vi "Host-Top-Level.vi"() -> ()   [LabVIEW 2017]
uses:
  <vilib>/rvi/interface/nirviMethod/nirviMethod.xnode
  <vilib>/FPGAPlugInAG/Dynamic/niLvFpga_Run_Dynamic.vi
panel:
  in  "Device address":string
  in  "Bitfile path":path
  in  "error in":errorcluster
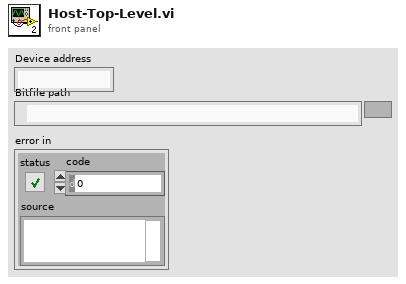
[diagram p1: front panel]
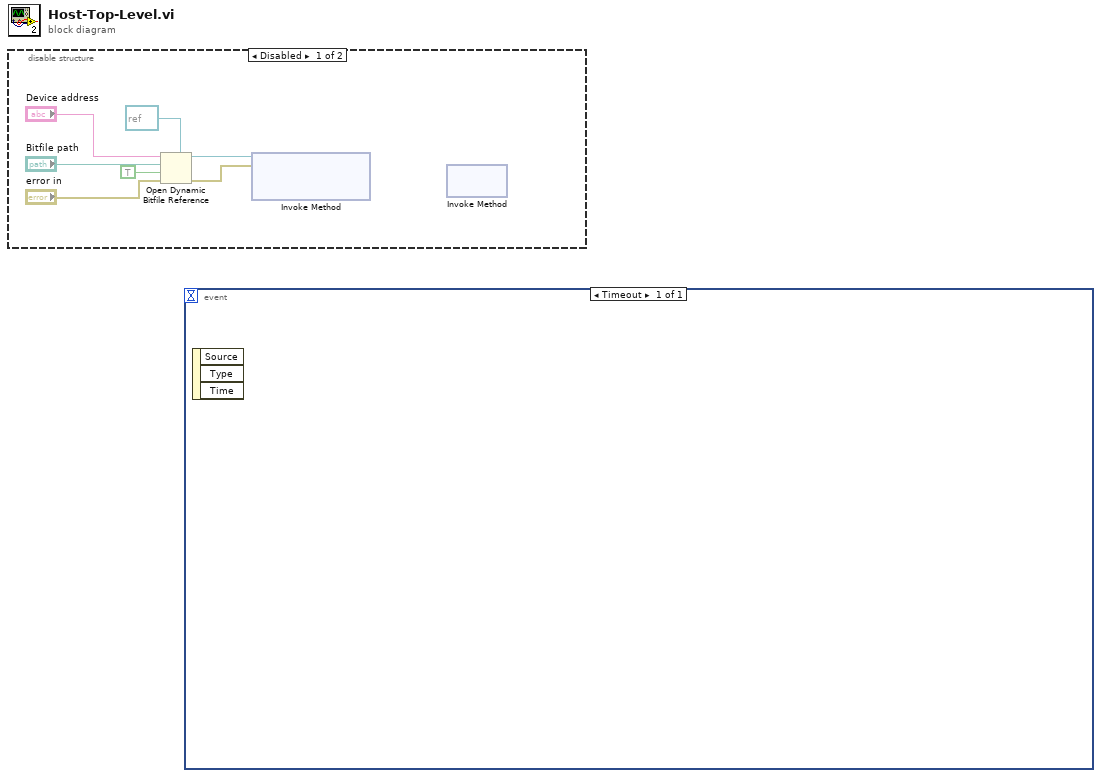
[diagram p0: block diagram]
diagram:
  n1 = disable-structure shown="Disabled" {
    frame Disabled {
      n2 = Open Dynamic Bitfile Reference(0:"Device address", 1:"Bitfile path", 2:TRUE ("Run When Loaded"), 3:"error in", 4:refnum<k20> refnum ("FPGA VI Reference Out")) -> (5:w2:refnum<k20>, 8:w1:errorcluster)
      n3 = xnode "Invoke Method"("FPGA VI Reference In"=w2, "error in"=w1) -> ()  [unwired: 1 in, 2 out]
      n4 = xnode "Invoke Method"() -> ()  [unwired: 2 in, 2 out]
    }
    frame Enabled {
    }
  }
  n5 = event shown="[0] Timeout" {
    selector: _ -> [_]
    dyn-events: _ -> [_]
    timeout: _ -> [_]
    event Timeout {
      n6 = event-data() -> ()  [unwired: 1 in, 3 out]
    }
  }
